vi "Test Color.vi"() -> ()   [LabVIEW 2017]
uses:
  <vilib>/addons/RealSense/libRealSense3.lvlib
  <vilib>/vision/NI_Vision_Development_Module.lvlib
panel:
  out "Image":T1(plugin-control)
  out "error out":errorcluster
  in  "stop":bool
  out "device count":i32
  # "All errors are #1, string is good"
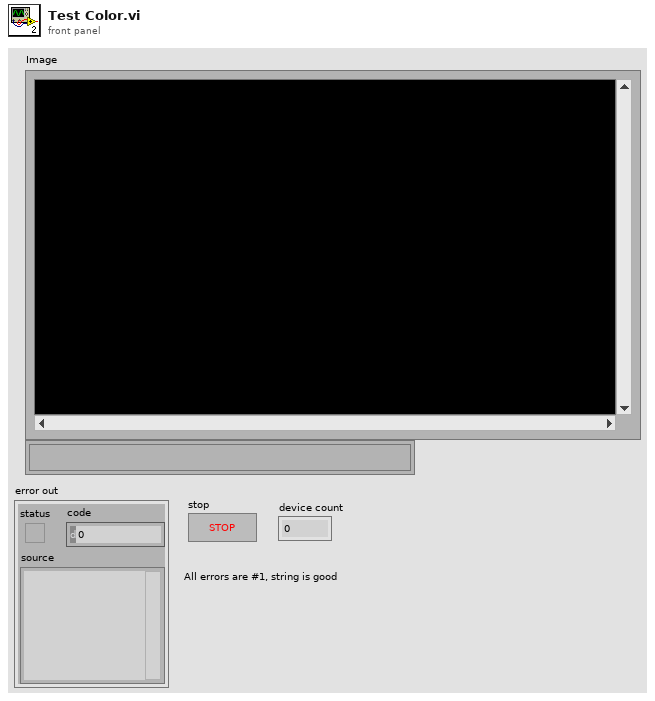
[diagram p1: front panel]
types:
  T1 = typedef "IMAQ Image.ctl" = refnum<image>
  T2 = typedef "Image Type" = u32
  T3 = cluster{"width":i32, "height":i32, "ppx":sgl, "ppy":sgl, "fx":sgl, "fy":sgl, "model":u32, "coeffs[0]":sgl, "coeffs[1]":sgl, "coeffs[2]":sgl, "coeffs[3]":sgl, "coeffs[4]":sgl}
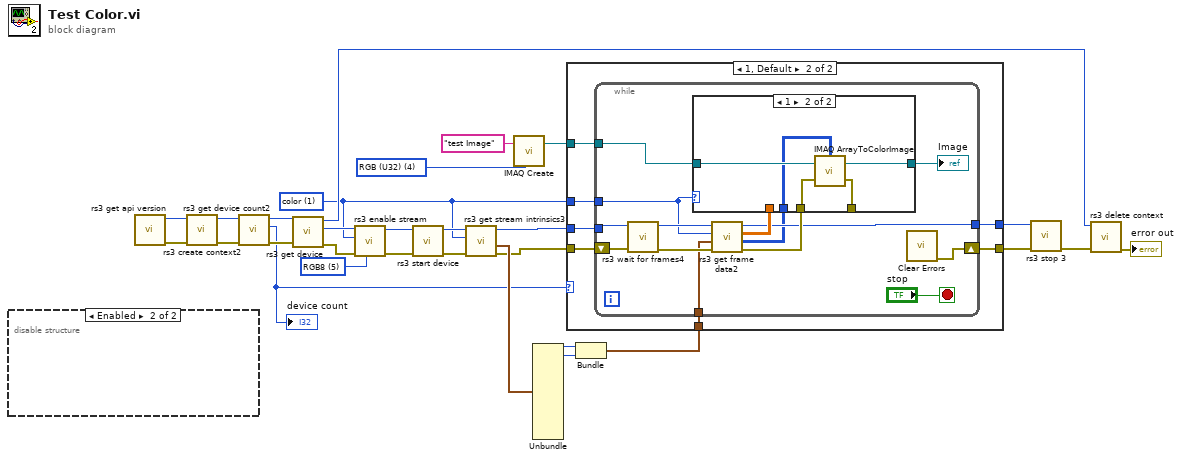
[diagram p0: block diagram]
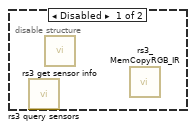
[diagram p2: hidden frame]
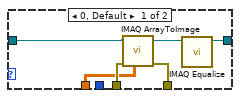
[diagram p4: hidden frame]
diagram:
  w2 = u16 5 items=["any", "Depth16", "Disparity16", "f32XYZ", "YUV", "RGB8", "BGR8", "RGBA8", "BGRA8", "Y8", "Y16", "Raw10", "Raw16", "Raw8"] ("format")
  w1 = u16 1 items=["depth", "color", "inf 1", "inf 2"] ("stream type")
  w4 = T2 4 items=["Grayscale (U8)", "Grayscale (I16)", "Grayscale (SGL)", "Complex (CSG)", "RGB (U32)", "HSL (U32)", "RGB (U64)", "Grayscale (U16)"] ("Image Type")
  n1 = disable-structure shown="Enabled" {
    frame Disabled {
      n2 = call <vilib>:"rs3 query sensors.vi"() -> ()  [unwired: 9 in, 3 out]
      n3 = call <vilib>:"rs3 get sensor info.vi"() -> ()  [unwired: 8 in, 4 out]
      n4 = call <vilib>:"rs3_MemCopyRGB_IR.vi"() -> ()  [unwired: 14 in, 2 out]
    }
    frame Enabled {
    }
  }
  n5 = call <vilib>:"rs3 get api version.vi"() -> ("error out"=w18:errorcluster, "version"=w29:i32)  [unwired: 10 in]
  n6 = call <vilib>:"rs3 create context2.vi"("error in (no error)"=w18, "version"=w29) -> ("error out"=w17:errorcluster, "context"=w28:u32)  [unwired: 8 in]
  n7 = call <vilib>:"rs3 get device count2.vi"("error in"=w17, "context"=w28) -> ("error out"=w16:errorcluster, "count"=w7:i32, "context"=w27:u32)  [unwired: 7 in]
  "device count" <- w7
  n8 = call <vilib>:"rs3 get device.vi"("error in"=w16, "context"=w27) -> ("error out"=w15:errorcluster, "device"=w26:u32, "context"=w19:u64)  [unwired: 7 in]
  n9 = call <vilib>:"rs3 enable stream.vi"("format"=w2, "error in"=w15, "stream type"=w1, "device"=w26) -> ("error out"=w14:errorcluster, "device"=w25:u32)  [unwired: 6 in]
  n10 = call <vilib>:"rs3 start device.vi"("error in"=w14, "device"=w25) -> ("error out"=w13:errorcluster, "device"=w24:u64)  [unwired: 8 in]
  n11 = call <vilib>:"rs3 get stream intrinsics3.vi"("error in (no error)"=w13, "stream type"=w1, "device in"=w24) -> ("error out"=w12:errorcluster, "intrin out"=w22:T3, "device out"=w23:u64)  [unwired: 6 in]
  n12 = call "IMAQ Create"("Image Name"="test Image", "Image Type"=w4) -> ("New Image"=w3:T1)  [unwired: 3 in, 1 out]
  n13 = Unbundle(w22) -> ("width"=w10:i32, "height"=w9:i32)  [unwired: 10 out]
  n14 = Bundle("width"=w10, "height"=w9) -> (w8:cluster{"width":i32, "height":i32})  [unwired: 1 in]
  n15 = case shown="1, Default" w7 {
    tunnel: w23 -> [w31 w38]
    tunnel: [w31 w37] -> w21
    tunnel: w12 -> [w30 w36]
    tunnel: [w30 w35] -> w11
    tunnel: w8 -> [_ w34]
    tunnel: w3 -> [_ w33]
    tunnel: w1 -> [_ w32]
    frame 0 {
    }
    frame 1, Default {
      n16 = while {
        tunnel: w38 -> [w51]
        tunnel: [w41] -> w37
        shift-right: [w49] -> w35
        shift-left: w36 -> [w50]
        tunnel: w34 -> [w45]
        tunnel: w33 -> [w47]
        tunnel: w32 -> [w40]
        stop <- "stop" stop-if-true
        n17 = call <vilib>:"rs3 wait for frames4.vi"("error in (no error)"=w50, "device in"=w51) -> ("error out"=w46:errorcluster, "device out"=w44:u64)  [unwired: 8 in]
        n18 = call <vilib>:"rs3 get frame data2.vi"("error in (no error)"=w46, "size"=w45, "stream type"=w40, "device in"=w44) -> ("error out"=w43:errorcluster, "2D Color Output"=w39:u32[][], "2D Depth Output"=w42:sgl[][], "device out"=w41:u64)  [unwired: 4 in]
        n19 = case shown="1" w40 {
          tunnel: w47 -> [w55 w63]
          tunnel: [w58 w62] -> w48
          tunnel: [w56 w61] -> _
          tunnel: w43 -> [w54 w60]
          tunnel: w42 -> [w53 _]
          tunnel: w39 -> [_ w59]
          frame 0, Default {
            n20 = call "IMAQ ArrayToImage"("Image Pixels (Float)"=w53, "error in (no error)"=w54, "Image"=w55) -> ("error out"=w56:errorcluster, "Image Out"=w57:T1)  [unwired: 7 in]
            n21 = call "IMAQ Equalize"("Image Src"=w57) -> ("Image Dst Out"=w58:T1)  [unwired: 9 in, 1 out]
          }
          frame 1 {
            n22 = call "IMAQ ArrayToColorImage"("Image Pixels (U32)"=w59, "Image"=w63, "error in (no error)"=w60) -> ("Image Out"=w62:T1, "error out"=w61:errorcluster)  [unwired: 2 in]
          }
        }
        "Image" <- w48
        n23 = call <vilib>:"Clear Errors.vi"() -> ("error out"=w49:errorcluster)  [unwired: 6 in, 1 out]
      }
    }
  }
  n24 = call <vilib>:"rs3 stop 3.vi"("error in (no error)"=w11, "device"=w21) -> ("error out"=w20:errorcluster)  [unwired: 8 in, 1 out]
  n25 = call <vilib>:"rs3 delete context.vi"("error in (no error)"=w20, "context"=w19) -> ("error out"=→"error out":errorcluster)  [unwired: 9 in]
